vi "Get Column Path.vi"(8 "error in (no error)":errorcluster, 9 "Column Name":string, 10 "Table path":string, 11 "Data.PG in":refnum<class "LV-Data.PGSQL.lvclass">) -> (0 "error out":errorcluster, 1 "Column Unit":string, 2 "Column Path":string, 3 "Data.PG out":refnum<class "LV-Data.PGSQL.lvclass">)   [LabVIEW 2019, in "LV-Data.PGSQL.lvclass"]
uses:
  LV-Data.PGSQL.lvclass
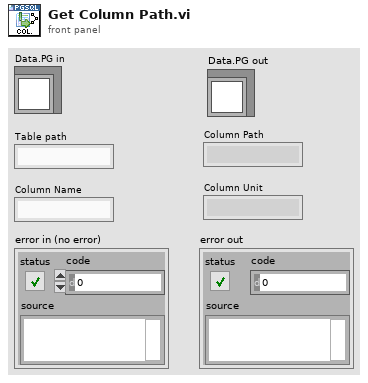
[diagram p1: front panel]
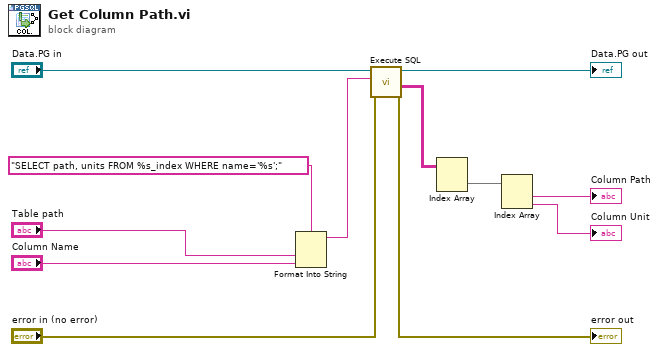
[diagram p0: block diagram]
diagram:
  n1 = Format Into String(format string="SELECT path, units FROM %s_index WHERE name='%s';", "Table path", "Column Name") -> (resulting string=w5:string)  [unwired: 2 in, 1 out]
  n2 = call "Execute SQL.vi"("error in"="error in (no error)", "SQL"=w5, "LV-Data.PGSQL"="Data.PG in") -> ("error out"=→"error out":errorcluster, "Result"=w1:string[][], "LV-Data.PGSQL out"=→"Data.PG out":refnum<class "LV-Data.PGSQL.lvclass">)  [unwired: 5 in, 1 out]
  n3 = Index Array(array=w1) -> (element=w6:string[])  [unwired: 2 in]
  n4 = Index Array(array=w6) -> (element #1=→"Column Path":string, element #2=→"Column Unit":string)  [unwired: 2 in]
